vi "Clone Registration AE.vi"(0 "Module ID":i32=-1, 1 "Action":T1=enum."Add Instance", 11 "error in (no error)":errorcluster) -> (3 "Instances Names":string[](array[string]), 4 "Module IDs":i32[](array[numeric]), 6 "First Module ID":i32, 8 "replaced":bool, 10 "Found?":bool, 13 "First?":bool, 14 "First? (all)":bool[](array[boolean]), 15 "error out":errorcluster)   [LabVIEW 2017, in "MQTT.lvlib" / "Clone Registration.lvlib"]
doc: "A registry (implemented as an Action Engine) to store all cloneable module instances. The Action Engine data is stored in a variant attribute table.\n\nOutput <b>First? </b> : We care which module instance was the first as the lifetime of the event references is bound to the lifetime of the module that created them (ie the first module instance). To avoid event references going bad we keep track of the first module and do not close it until safe to do so (ie when all other instances have closed).\n\nIf the first instance is closed whilst others are still running we effectively set that instance to idle. We deregister for all requests except STOP ALL.\n_____\nBased on Delacor QMH Project Template 3.1.0.34."
uses:
  Clone Registration.lvlib
  Action--enum.ctl
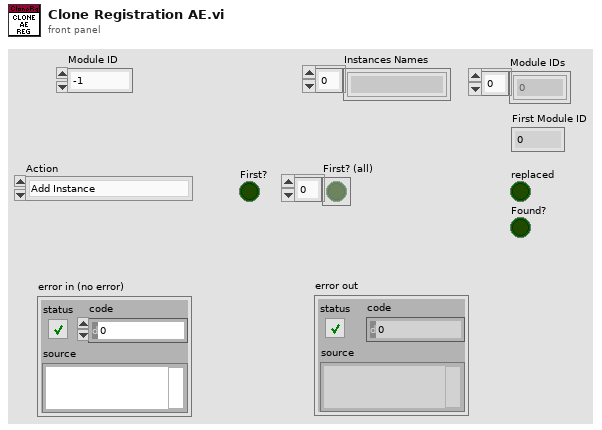
[diagram p1: front panel]
types:
  T1 = typedef "MQTT.lvlib/Clone Registration.lvlib/Action--enum.ctl" = enum16{"Init", "Add Instance", "Remove Instance", "List Instances", "Is First?"}
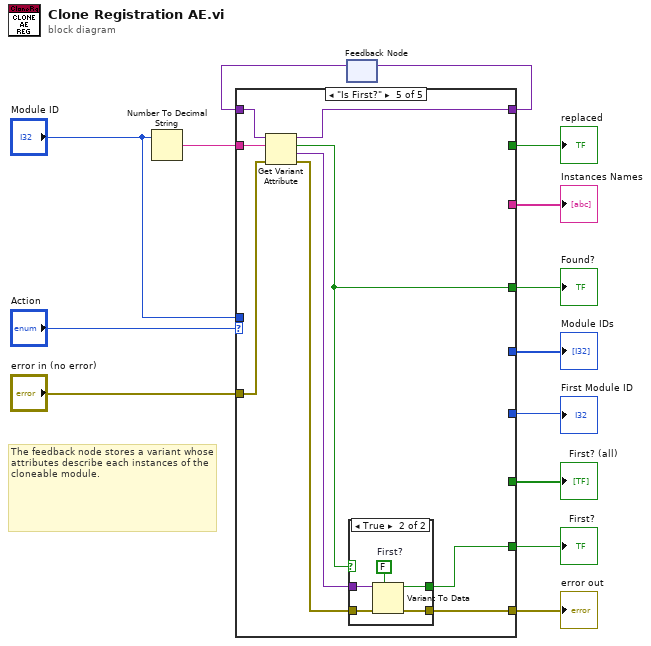
[diagram p0: block diagram]
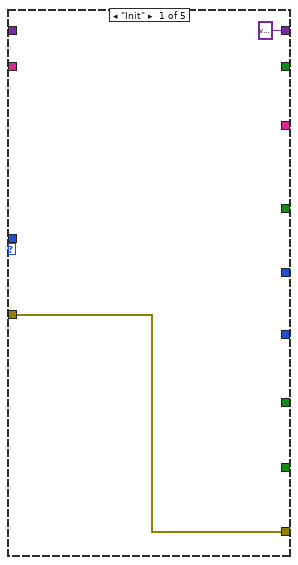
[diagram p2: hidden frame]
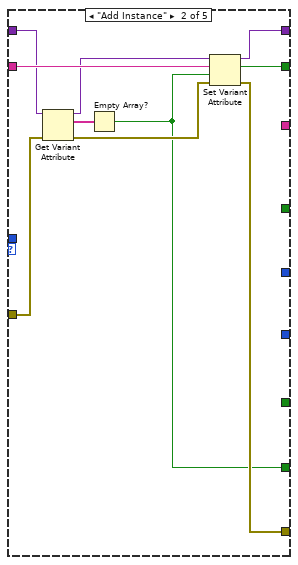
[diagram p3: hidden frame]
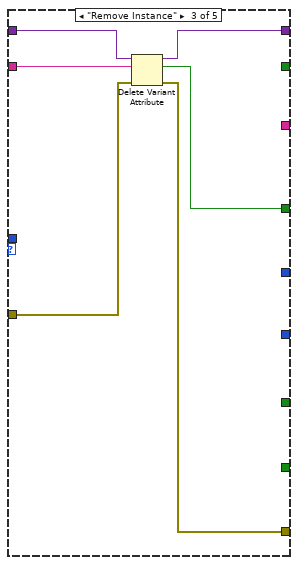
[diagram p4: hidden frame]
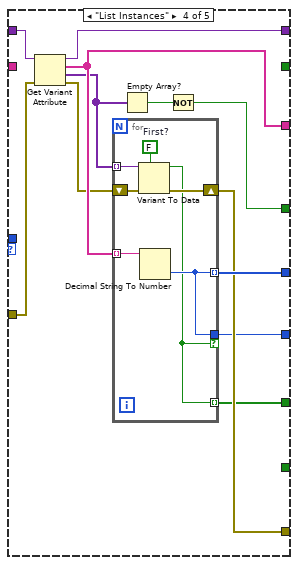
[diagram p5: hidden frame]
diagram:
  # "The feedback node stores a variant whose attributes describe each instances of the cloneable module."
  n1 = Number To Decimal String(number="Module ID") -> (decimal integer string=w13:string)  [unwired: 1 in]
  n2 = feedback #1() -> (w11:variant)  [unwired: 1 in]
  n3 = case shown="\"Is First?\"" "Action" {
    tunnel: w11 -> [_ w23 w32 w44 w60]
    tunnel: [variant w26 w31 w43 w59] -> w10
    tunnel: w13 -> [_ w25 w30 _ w54]
    tunnel: [_ w24 _ _ _] -> w9
    tunnel: [_ _ w29 w41 w52] -> w8
    tunnel: "Module ID" -> [_ _ _ _ _]
    tunnel: [_ _ _ w40 _] -> w7
    tunnel: [_ _ _ w39 _] -> w6
    tunnel: [_ _ _ w34 _] -> w5
    tunnel: "error in (no error)" -> [w15 w20 w28 w37 w57]
    tunnel: [w15 w18 w27 w35 w55] -> w3
    tunnel: [_ _ _ w33 _] -> w2
    tunnel: [_ w17 _ _ w53] -> w1
    frame "Init" {
    }
    frame "Add Instance" {
      n4 = Get Variant Attribute(Variant=w23, error in=w20) -> (duplicate Variant=w22:variant, names=w21:string[], error out=w19:errorcluster)  [unwired: 2 in, 1 out]
      n5 = Empty Array?(array=w21) -> (empty?=w17:bool)
      n6 = Set Variant Attribute(Variant=w22, name=w25, value=w17, error in=w19) -> (Variant out=w26:variant, replaced=w24:bool, error out=w18:errorcluster)
    }
    frame "Remove Instance" {
      n7 = Delete Variant Attribute(4:w28, 6:w30, 7:w32) -> (0:w27:errorcluster, 2:w29:bool, 3:w31:variant)
    }
    frame "List Instances" {
      n8 = Get Variant Attribute(Variant=w44, error in=w37) -> (duplicate Variant=w43:variant, names=w39:string[], values=w38:variant[], error out=w36:errorcluster)  [unwired: 2 in]
      n9 = for {
        tunnel: w39 -> [w51] mode=indexing
        tunnel: [w46] -> w40 mode=indexing
        tunnel: w38 -> [w50] mode=indexing
        shift-right: [w47] -> w35
        shift-left: w36 -> [w48]
        tunnel: [w45] -> w34 mode=indexing
        tunnel: [w46] -> w33 if=w45
        w49 = FALSE  # First?
        n10 = Variant To Data(error in=w48, type=w49, Variant=w50) -> (data=w45:bool, error out=w47:errorcluster)
        n11 = Decimal String To Number(string=w51) -> (number=w46:i32)  [unwired: 2 in, 1 out]
      }
      n12 = Empty Array?(array=w38) -> (empty?=w42:bool)
      n13 = Not(x=w42) -> (.not. x?=w41:bool)
    }
    frame "Is First?" {
      n14 = Get Variant Attribute(Variant=w60, name=w54, error in=w57) -> (duplicate Variant=w59:variant, found=w52:bool, value=w58:variant, error out=w56:errorcluster)  [unwired: 1 in]
      n15 = case shown="True" w52 {
        tunnel: w58 -> [_ w66]
        tunnel: w56 -> [w61 w65]
        tunnel: [w61 w64] -> w55
        tunnel: [_ w62] -> w53
        frame False {
        }
        frame True {
          w63 = FALSE  # First?
          n16 = Variant To Data(error in=w65, type=w63, Variant=w66) -> (data=w62:bool, error out=w64:errorcluster)
        }
      }
    }
  }
  "replaced" <- w9
  "Found?" <- w8
  "Module IDs" <- w7
  "Instances Names" <- w6
  "First? (all)" <- w5
  "error out" <- w3
  "First Module ID" <- w2
  "First?" <- w1
  n17 = feedback-in #1(w10) -> ()
